vi "EdgeCutPlaneIntersect.vi"(10 "CuttingZ":sgl, 11 "Line3D":T2) -> (2 "Intersect?":bool, 3 "IntersectPoint":T1)   [LabVIEW 2014]
uses:
  TypeDefs/Line3D.ctl
  TypeDefs/Point3D.ctl
  TypeDefs/Point2D.ctl
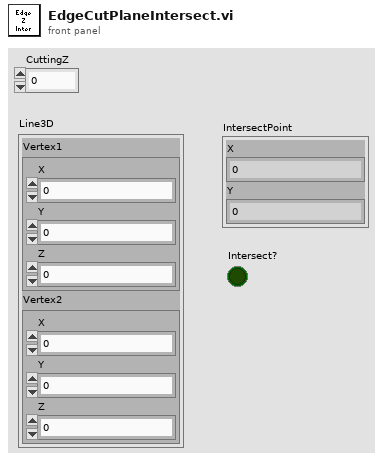
[diagram p1: front panel]
types:
  T1 = typedef "Point2D.ctl" = cluster{"X":sgl, "Y":sgl}
  T2 = typedef "Line3D.ctl" = cluster{"Vertex1":T3, "Vertex2":T3}
  T3 = typedef "Point3D.ctl" = cluster{"X":sgl, "Y":sgl, "Z":sgl}
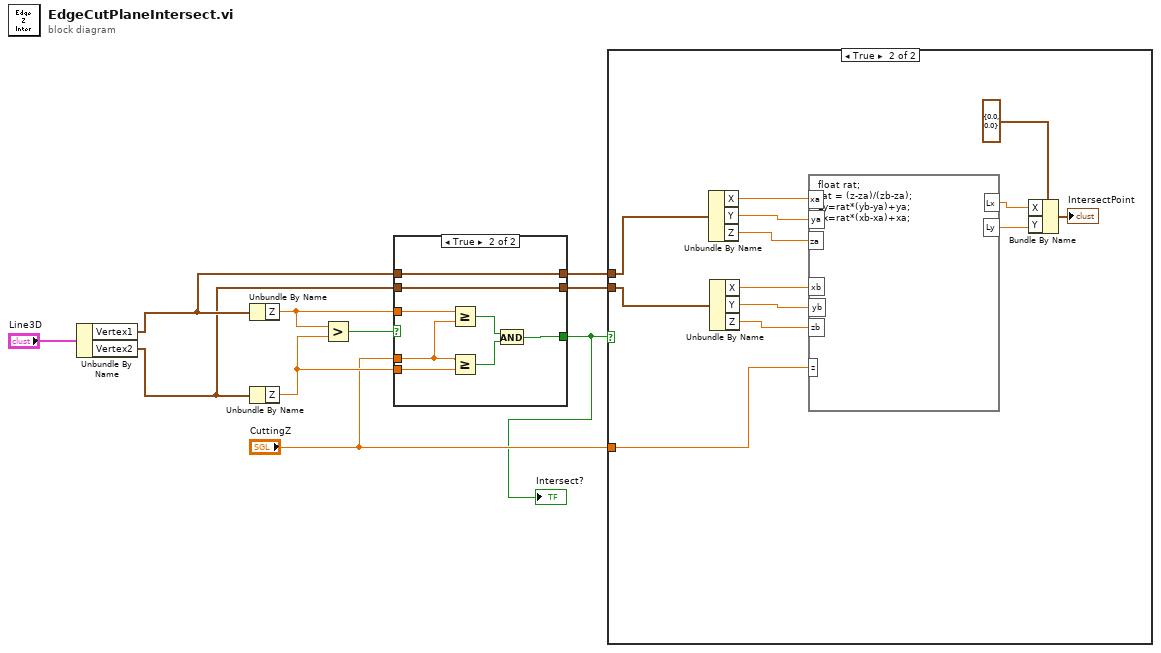
[diagram p0: block diagram]
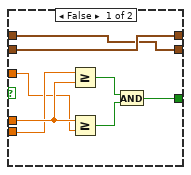
[diagram p3: hidden frame]
diagram:
  n1 = Unbundle By Name("Line3D") -> ("Vertex1"=w5:T3, "Vertex2"=w4:T3)
  n2 = Unbundle By Name(w5) -> ("Z"=w8:sgl)
  n3 = Unbundle By Name(w4) -> ("Z"=w7:sgl)
  n4 = Greater?(x=w8, y=w7) -> (0:w9:bool)
  n5 = case shown="True" w9 {
    tunnel: w8 -> [w14 w26]
    tunnel: "CuttingZ" -> [w16 w25]
    tunnel: w7 -> [w15 w24]
    tunnel: [w13 w21] -> w1
    tunnel: [w12 w20] -> w6
    tunnel: w5 -> [w11 w20]
    tunnel: w4 -> [w12 w19]
    tunnel: [w11 w19] -> w3
    frame False {
      n6 = Greater Or Equal?(x=w15, y=w16) -> (x >= y?=w18:bool)
      n7 = Greater Or Equal?(x=w16, y=w14) -> (x >= y?=w17:bool)
      n8 = And(x=w18, y=w17) -> (x .and. y?=w13:bool)
    }
    frame True {
      n9 = Greater Or Equal?(x=w26, y=w25) -> (x >= y?=w23:bool)
      n10 = Greater Or Equal?(x=w25, y=w24) -> (x >= y?=w22:bool)
      n11 = And(x=w23, y=w22) -> (x .and. y?=w21:bool)
    }
  }
  "Intersect?" <- w1
  n12 = case shown="True" w1 {
    tunnel: w6 -> [_ w39]
    tunnel: w3 -> [_ w38]
    tunnel: "CuttingZ" -> [_ w31]
    frame False {
    }
    frame True {
      n13 = Unbundle By Name(w39) -> ("X"=w37:sgl, "Y"=w36:sgl, "Z"=w35:sgl)
      n14 = Unbundle By Name(w38) -> ("X"=w34:sgl, "Y"=w33:sgl, "Z"=w32:sgl)
      n15 = formula code="float rat;\nrat = (z-za)/(zb-za);\nLy=rat*(yb-ya)+ya;\nLx=rat*(xb-xa)+xa;"("xa"=w37, "ya"=w36, "za"=w35, "xb"=w34, "yb"=w33, "zb"=w32, "z"=w31) -> ("Ly"=w28:dbl, "Lx"=w29:dbl)
      n16 = Bundle By Name(cluster=T1 {"X"=0.0, "Y"=0.0} ("Point2D"), "X"=w29, "Y"=w28) -> (→"IntersectPoint":T1)
    }
  }
